vi "Number of Poly Order in Zeta Function.vi"(11 "x":cdb) -> (3 "n":i32)   [LabVIEW 2020, in "NI_Gmath.lvlib"]
uses:
  <vilib>/gmath/NI_Gmath.lvlib
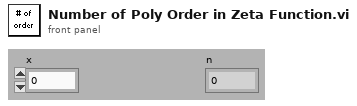
[diagram p1: front panel]
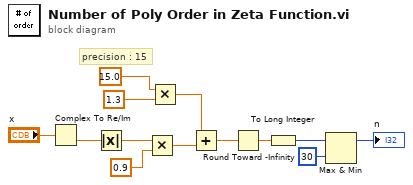
[diagram p0: block diagram]
diagram:
  # "precision : 15"
  n1 = Complex To Re/Im(x + iy="x") -> (y=w12:dbl)  [unwired: 1 out]
  n2 = Absolute Value(x=w12) -> (abs(x)=w9:dbl)
  n3 = Multiply(x=w9, y=0.9) -> (x*y=w7:dbl)
  n4 = Multiply(x=15.0, y=1.3) -> (x*y=w6:dbl)
  n5 = Add(x=w6, y=w7) -> (x+y=w5:dbl)
  n6 = Round Toward -Infinity(1:w5) -> (0:w4:dbl)
  n7 = To Long Integer(number=w4) -> (32bit integer=w3:i32)
  n8 = Max & Min(x=w3, y=30) -> (max(x,y)=→"n":i32)  [unwired: 1 out]
